vi "Post-Build Action Helper.vi"(8 "error in (no error)":errorcluster, 10 "build specification name":string, 11 "destination path":path) -> (0 "error out":errorcluster)   [LabVIEW 2025, in "I2C Bus Monitor.lvclass"]
uses:
  I2C Bus Monitor.lvclass
  I2C Bus Monitor.lvclass/I2C Bus Monitor.ctl
  <vilib>/Utility/sysdir.llb/System Directory Type.ctl
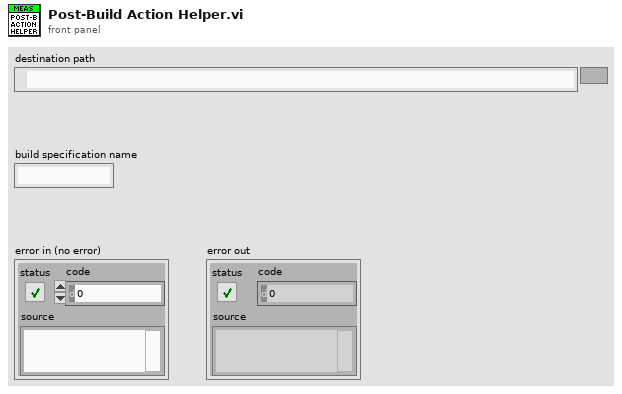
[diagram p1: front panel]
types:
  T1 = typedef "System Directory Type.ctl" = i32
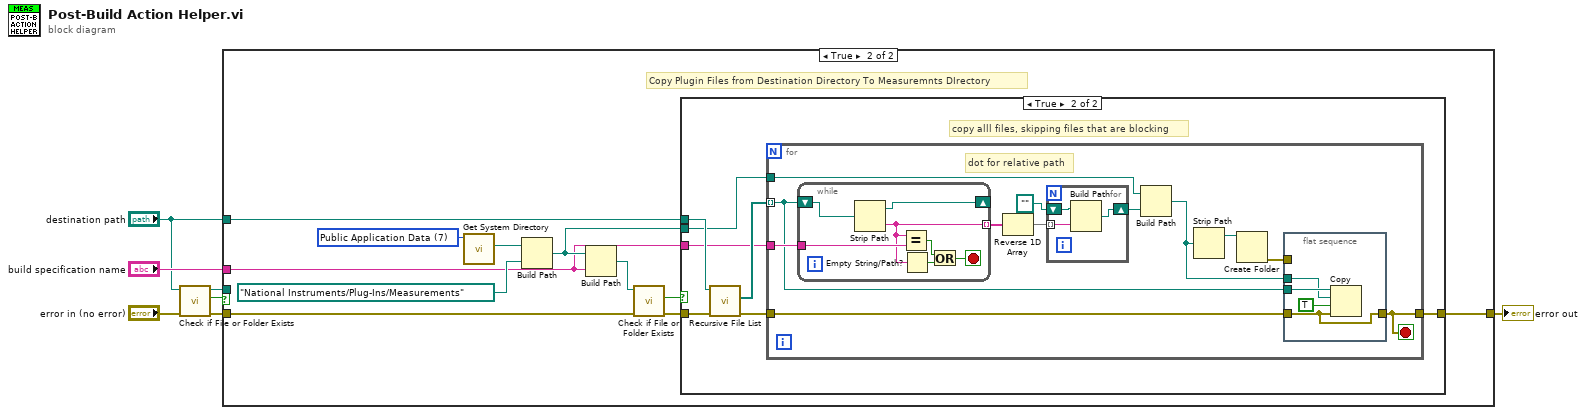
[diagram p0: block diagram]
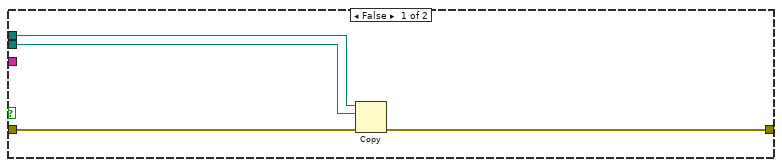
[diagram p3: hidden frame]
diagram:
  n1 = call <vilib>:"Check if File or Folder Exists.vi"("error in (no error)"="error in (no error)", "path"="destination path") -> ("error out"=w2:errorcluster, "file or folder exists?"=w4:bool, "dup path"=w5:path)  [unwired: 7 in]
  n2 = case shown="True" w4 {
    tunnel: w2 -> [w8 w16]
    tunnel: [w8 w10] -> w3
    tunnel: w5 -> [_ _]
    tunnel: "destination path" -> [_ w11]
    tunnel: "build specification name" -> [_ w9]
    frame False {
    }
    frame True {
      w19 = T1 7 items=["User Home"=0, "User Desktop"=1, "User Documents"=2, "User Application Data"=3, "User Preferences"=4, "User Temporary"=5, "Public Documents"=6, "Public Application Data"=7, "Public Preferences"=8, "Public Cache"=13, "System Core Libraries"=9, "System Installed Libraries"=10, "Application Files"=11, "Boot Volume Root"=12] ("system directory type")
      # "Copy Plugin Files from Destination Directory To Measuremnts DIrectory"
      n3 = call <vilib>:"Get System Directory.vi"("system directory type"=w19) -> ("system directory"=w18:path)  [unwired: 10 in]
      n4 = Build Path(base path=w18, name or relative path=path "National Instruments/Plug-Ins/Measurements") -> (appended path=w12:path)
      n5 = Build Path(base path=w12, name or relative path=w9) -> (appended path=w15:path)
      n6 = call <vilib>:"Check if File or Folder Exists.vi"("error in (no error)"=w16, "path"=w15) -> ("error out"=w14:errorcluster, "file or folder exists?"=w13:bool)  [unwired: 7 in, 1 out]
      n7 = case shown="True" w13 {
        tunnel: w14 -> [w20 w28]
        tunnel: w12 -> [w23 w26]
        tunnel: w11 -> [w22 w27]
        tunnel: [w21 w24] -> w10
        tunnel: w9 -> [_ w25]
        frame False {
          n8 = Copy(8:w20, 10:w23, 11:w22) -> (0:w21:errorcluster)  [unwired: 2 in, 2 out]
        }
        frame True {
          # "copy alll files, skipping files that are blocking"
          n9 = call <vilib>:"Recursive File List.vi"("error in (no error)"=w28, "Folder Path"=w27) -> ("error out"=w29:errorcluster, "All Files in Dir"=w30:path[])  [unwired: 5 in, 3 out]
          n10 = for {
            tunnel: w30 -> [w36] mode=indexing
            tunnel: w25 -> [w42]
            tunnel: w26 -> [w37]
            tunnel: w29 -> [w32]
            tunnel: [w31] -> w24
            stop <- w31 stop-if-true
            # "dot for relative path"
            n11 = while {
              tunnel: [w52] -> w39 mode=indexing
              tunnel: w42 -> [w55]
              shift-right: [w50] -> _
              shift-left: w36 -> [w56]
              stop <- w53 stop-if-true
              n12 = Strip Path(path=w56) -> (stripped path=w50:path, name=w52:string)
              n13 = Equal?(x=w52, y=w55) -> (x = y?=w54:bool)
              n14 = Empty String/Path?(string/path=w52) -> (empty?=w51:bool)
              n15 = Or(x=w54, y=w51) -> (x .or. y?=w53:bool)
            }
            n16 = Reverse 1D Array(array=w39) -> (reversed array=w41:string[])
            n17 = for {
              tunnel: w41 -> [w49] mode=indexing
              shift-right: [w47] -> w38
              shift-left: path "" ("appended path") -> [w48]
              n18 = Build Path(base path=w48, name or relative path=w49) -> (appended path=w47:path)
            }
            n19 = Build Path(base path=w37, name or relative path=w38) -> (appended path=w35:path)
            n20 = Strip Path(path=w35) -> (stripped path=w34:path)  [unwired: 1 out]
            n21 = Create Folder(path (use dialog)=w34) -> (error out=w33:errorcluster)  [unwired: 2 in, 2 out]
            n22 = flat-sequence {
              tunnel: w36 -> [w46]
              tunnel: [w43] -> w31
              tunnel: w35 -> [w44]
              tunnel: w33 -> [_]
              tunnel: w32 -> [w43]
              frame #0 {
                n23 = Copy(8:w43, 9:TRUE ("overwrite (F)"), 10:w44, 11:w46) -> ()  [unwired: 1 in, 3 out]
              }
            }
          }
        }
      }
    }
  }
  "error out" <- w3
